vi "Actor Core.vi"(8 "error in":errorcluster, 11 "View Manager In":refnum<class "View Manager.lvclass">=refnum) -> (0 "error out":errorcluster, 3 "Actor out":refnum<class "Actor.lvclass">)   [LabVIEW 2017, in "View Manager.lvlib" / "View Manager.lvclass"]
doc: "(<B>Filename</B>: Actor Framework.lvlib:Actor.lvclass:Actor Core.vi)\n\nReceives messages to the actor, reacts to them, and initiates any error handling that may shut the actor down.\n\nDescendant classes may override this VI to append parallel tasks for the actor to complete while it handles messages. Overrides use the Call Parent Method node.\n\n<License>\nCopyright © 2017 Composed Systems, LLC | All rights reserved\nwww.composed.io\n\nAuthor: Ethan Stern <ethan.stern@composed.io>\n\nThis software is provided \"AS IS\" WITHOUT WARRANTIES, either express or implied, AND IS FOR EDUCATIONAL PURPOSES ONLY.\n</License>"
uses:
  View Manager.lvclass
  <vilib>/gpm_packages/@cs/mva-viewable/Source/IViewable/ProtectedSubpanel/ProtectedSubpanel.lvclass
  <vilib>/event_ctls.llb/lveventtype.ctl
  <vilib>/gpm_packages/@cs/mva-viewable/Source/ActorEvents/IEventAggregator/IEventAggregator.lvclass
  <vilib>/gpm_packages/@cs/mva-core/Source/IObserver/IObserver/IObserver.lvclass
  View Manager Messages/Login Msg/Login Msg.lvclass
  View Manager Messages/Logout Msg/Logout Msg.lvclass
  <vilib>/gpm_packages/@cs/mva-core/Source/SubscriptionPolicy/BasicSubscription/BasicSubscription.lvclass
  User Manager Model/Type Definitions/Successful Login Information.ctl
  User Manager Model/Type Definitions/User Manager Application Types.lvlib
  User Manager Model/Type Definitions/User Levels.ctl
  C:/Program Files/National Instruments/LabVIEW 2017/vi.lib/gpm_packages/@cs/mva-core/Source/IObserver/IObserver/IObserver.lvclass
  C:/Program Files/National Instruments/LabVIEW 2017/vi.lib/ActorFramework/Actor/Actor.lvclass
  C:/Program Files/National Instruments/LabVIEW 2017/vi.lib/gpm_packages/@cs/mva-core/Source/IMediator/ISubscriptionPolicy/ISubscriptionPolicy.lvclass
  C:/Program Files/National Instruments/LabVIEW 2017/vi.lib/gpm_packages/@cs/transport/Source/Concrete/ActorMessageTransport/Notification Msg/Notification Msg.lvclass
  C:/Program Files/National Instruments/LabVIEW 2017/vi.lib/gpm_packages/@cs/actor-framework-messages/Source/RoundTripMessage/RoundTripMessage.lvclass
  C:/Program Files/National Instruments/LabVIEW 2017/vi.lib/ActorFramework/Message/Message.lvclass
  <vilib>/ActorFramework/Actor/Actor.lvclass
panel:
  in  "Logout":bool
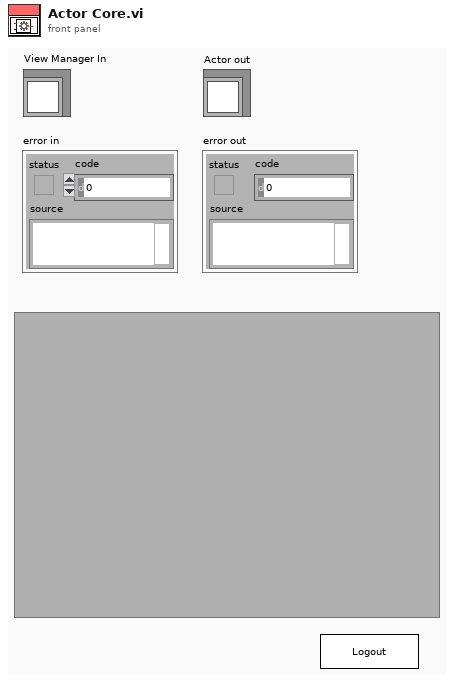
[diagram p1: front panel]
types:
  T1 = typedef "User Manager Application Types.lvlib/Successful Login Information.ctl" = cluster{"Username":string, "User Level":T2, "User Levels In This Society":T2[]}
  T2 = typedef "User Manager Application Types.lvlib/User Levels.ctl" = cluster{"Rank":i32, "Title":string}
  T3 = typedef "lveventtype.ctl" = enum32{"Null", "Timeout", "Annotation Menu Selection", "Annotation Menu Selection?", "App Instance Close", "App Instance Close?", "Autoscale Range Change", "Bookmark Info Change", "Cell Edit", "Cell Edit?", "Cursor Grab", "Cursor Grab?", "Cursor Menu Selection", "Cursor Menu Selection?", "Cursor Move", "Cursor Release", "Data Change", "Direction Change", "Display State Change", "Drag Ended", "Drag Enter", "Drag Leave", "Drag Over", "Drag Source Update", "Drag Starting", "Drag Starting?", "Drop", "Exec State Change", "Key Down", "Key Down?", "Key Repeat", "Key Repeat?", "Key Up", "Listbox Double Click", "Menu Activation?", "Menu Selection (App)", "Menu Selection? (App)", "Menu Selection (User)", "Mouse Down", "Mouse Down?", "Mouse Enter", "Mouse Leave", "Mouse Move", "Mouse Up", "Mouse Wheel", "NI Security User Change (App)", "Pane Size", "Panel Close", "Panel Close?", "Panel Resize", "Plot Attribute Change", "Scale Range Change", "Shortcut Menu Activation?", "Shortcut Menu Selection (App)", "Shortcut Menu Selection? (App)", "Shortcut Menu Selection (User)", "Tree Double Click", "Tree Drag", "Tree Drag?", "Tree Drop", "Tree Drop?", "Tree Item Close", "Tree Item Close?", "Tree Item Open", "Tree Item Open?", "User Event", "Value Change"}
  T4 = typedef "IViewable.lvlib/ProtectedSubpanel.lvclass/Protected Subpanel Reference.ctl" = refnum<data-value>
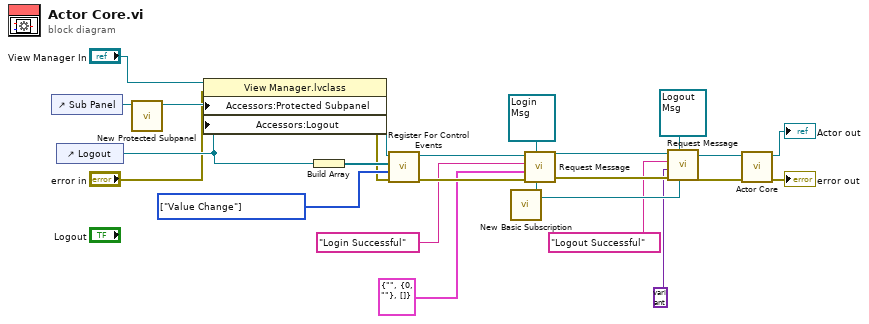
[diagram p0: block diagram]
diagram:
  w20 = T3[] [enum."Value Change"] items=["Null", "Timeout", "Annotation Menu Selection", "Annotation Menu Selection?", "App Instance Close", "App Instance Close?", "Autoscale Range Change", "Bookmark Info Change", "Cell Edit", "Cell Edit?", "Cursor Grab", "Cursor Grab?", "Cursor Menu Selection", "Cursor Menu Selection?", "Cursor Move", "Cursor Release", "Data Change", "Direction Change", "Display State Change", "Drag Ended", "Drag Enter", "Drag Leave", "Drag Over", "Drag Source Update", "Drag Starting", "Drag Starting?", "Drop", "Exec State Change", "Key Down", "Key Down?", "Key Repeat", "Key Repeat?", "Key Up", "Listbox Double Click", "Menu Activation?", "Menu Selection (App)", "Menu Selection? (App)", "Menu Selection (User)", "Mouse Down", "Mouse Down?", "Mouse Enter", "Mouse Leave", "Mouse Move", "Mouse Up", "Mouse Wheel", "NI Security User Change (App)", "Pane Size", "Panel Close", "Panel Close?", "Panel Resize", "Plot Attribute Change", "Scale Range Change", "Shortcut Menu Activation?", "Shortcut Menu Selection (App)", "Shortcut Menu Selection? (App)", "Shortcut Menu Selection (User)", "Tree Double Click", "Tree Drag", "Tree Drag?", "Tree Drop", "Tree Drop?", "Tree Item Close", "Tree Item Close?", "Tree Item Open", "Tree Item Open?", "User Event", "Value Change"] ("Registration Types")
  n1 = control-ref of="Sub Panel"() -> (w22:refnum<vi>)
  n2 = control-ref of="Logout"() -> (w4:refnum<vi>)
  n3 = call <vilib>:"New Protected Subpanel.vi"("SubPnl Refnum"=w22) -> ("Protected Subpanel"=w5:T4)  [unwired: 9 in, 1 out]
  n4 = property class="View Manager.lvclass"(reference="View Manager In", error in="error in", "Accessors:Protected Subpanel"=w5, "Accessors:Logout"=w4) -> (reference out=w3:refnum<class "View Manager.lvclass">, error out=w1:errorcluster)
  n5 = Build Array(w4) -> (w21:refnum<vi>[])
  n6 = call <vilib>:"Register For Control Events.vi"("error in (no error)"=w1, "Registration Types"=w20, "Control Refnums"=w21, "IEventAggregator In"=w3) -> ("error out"=w18:errorcluster, "IEventAggregator Out"=w19:refnum<class "IEventAggregator.lvclass">)  [unwired: 6 in]
  n7 = call <vilib>:"New Basic Subscription.vi"() -> ("BasicSubscription Out"=w10:refnum<class "BasicSubscription.lvclass">)  [unwired: 11 in]
  n8 = call <vilib>:"Request Message.vi"("Configured SubscriptionPolicy"=w10, "Desired Notification Msg"=refnum<class "Login Msg.lvclass"> refnum ("View Manager.lvlib:Login Msg.lvclass"), "error in (no error)"=w18, "Data Type"=T1 {"Username"="", "User Level"={"Rank"=0, "Title"=""}, "User Levels In This Society"=[]}, "Datum Name"="Login Successful", "IObserver in"=w19) -> ("error out"=w16:errorcluster, "IObserver out"=w17:refnum<class "IEventAggregator.lvclass">)  [unwired: 3 in, 1 out]
  n9 = call <vilib>:"Request Message.vi"("Configured SubscriptionPolicy"=w10, "Desired Notification Msg"=refnum<class "Logout Msg.lvclass"> refnum ("View Manager.lvlib:Logout Msg.lvclass"), "error in (no error)"=w16, "Data Type"=variant, "Datum Name"="Logout Successful", "IObserver in"=w17) -> ("error out"=w14:errorcluster, "IObserver out"=w15:refnum<class "IEventAggregator.lvclass">)  [unwired: 3 in, 1 out]
  n10 = call-parent "Actor Core.vi"("error in"=w14, "IViewable In"=w15) -> ("error out"=→"error out":errorcluster, "Actor out"=→"Actor out":refnum<class "Actor.lvclass">)  [unwired: 8 in]
